vi "Stop TCS.vi"(8 "error in (no error)":errorcluster, 11 "AutoExp in":refnum<class "AutoExp.lvclass">) -> (0 "error out":errorcluster, 3 "AutoExp out":refnum<class "AutoExp.lvclass">)   [LabVIEW 2018, in "AutoExp.lvclass"]
uses:
  AutoExp.lvclass
  AutoExp.lvclass/AutoExp.ctl
  TCS/TCS.lvclass
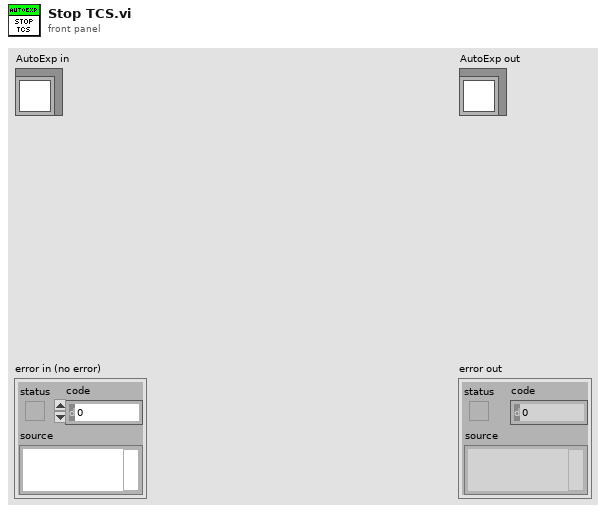
[diagram p1: front panel]
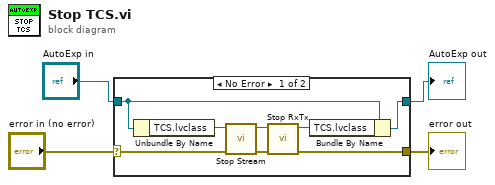
[diagram p0: block diagram]
diagram:
  n1 = case shown="No Error" "error in (no error)" {
    selector: "error in (no error)" -> [w5 w14]
    tunnel: [w6 w14] -> w3
    tunnel: [w9 w13] -> w1
    tunnel: "AutoExp in" -> [w10 w13]
    frame No Error {
      n2 = Unbundle By Name(w10) -> ("TCS.lvclass"=w12:refnum<class "TCS.lvclass">)
      n3 = call "Stop Stream.vi"("error in (no error)"=w5, "TCS in"=w12) -> ("error out"=w7:errorcluster, "TCS out"=w11:refnum<class "TCS.lvclass">)  [unwired: 8 in]
      n4 = call "Stop RxTx.vi"("error in (no error)"=w7, "TCS in"=w11) -> ("error out"=w6:errorcluster, "TCS out"=w8:refnum<class "TCS.lvclass">)  [unwired: 8 in]
      n5 = Bundle By Name(cluster=w10, "TCS.lvclass"=w8) -> (w9:refnum<class "AutoExp.lvclass">)
    }
    frame Error {
    }
  }
  "error out" <- w3
  "AutoExp out" <- w1
